vi "Format Module Name.vi"(11 "Module Path":string) -> (3 "Formatted Module Path":string)   [LabVIEW 2017, in "Routing and Faulting System Explorer.lvlib"]
uses:
  Routing and Faulting System Explorer.lvlib
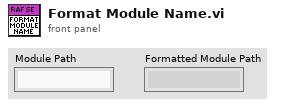
[diagram p1: front panel]
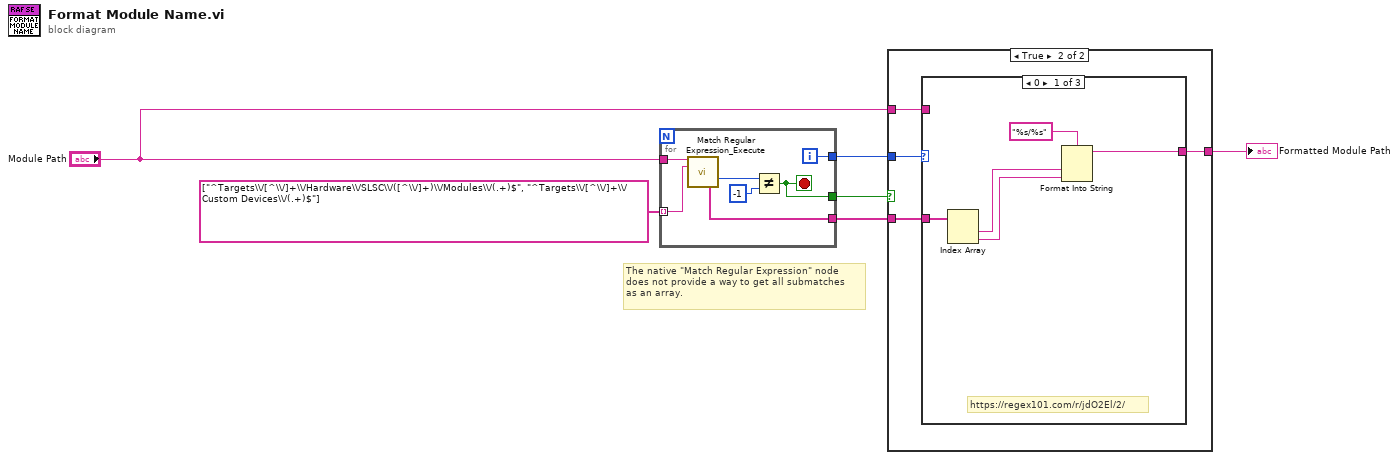
[diagram p0: block diagram]
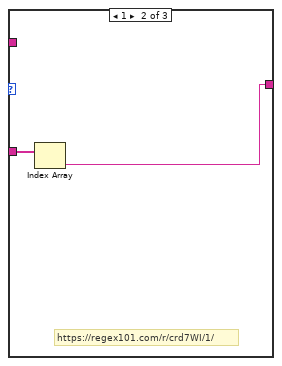
[diagram p3: hidden frame]
diagram:
  # "The native \"Match Regular Expression\" node\ndoes not provide a way to get all submatches\nas an array."
  n1 = for {
    tunnel: "Module Path" -> [w11]
    tunnel: string[] ["^Targets\\/[^\\/]+\\/Hardware\\/SLSC\\/([^\\/]+)\\/Modules\\/(.+)$", "^Targets\\/[^\\/]+\\/Custom Devices\\/(.+)$"] -> [w10] mode=indexing
    tunnel: [w12] -> w2
    tunnel: [w8] -> w4
    tunnel: [w7] -> w3
    i -> [w12]
    stop <- w7 stop-if-true
    n2 = call <vilib>:"Match Regular Expression_Execute.vi"("input string"=w11, "regular expression"=w10) -> ("whole match offset"=w9:i32, "matched substrings"=w8:string[])  [unwired: 8 in, 4 out]
    n3 = Not Equal?(x=w9, y=-1) -> (x != y?=w7:bool)
  }
  n4 = case shown="True" w3 {
    tunnel: w2 -> [_ w18]
    tunnel: w4 -> [_ w17]
    tunnel: "Module Path" -> [w14 w16]
    tunnel: [w14 w15] -> w5
    frame False {
    }
    frame True {
      n5 = case shown="0" w18 {
        tunnel: w17 -> [w23 w25 _]
        tunnel: w16 -> [_ _ w26]
        tunnel: [w19 w24 w26] -> w15
        frame 0 {
          # "https://regex101.com/r/jdO2El/2/"
          n6 = Index Array(array=w23) -> (element #1=w21:string, element #2=w20:string)  [unwired: 2 in]
          n7 = Format Into String(format string="%s/%s", w21, w20) -> (resulting string=w19:string)  [unwired: 2 in, 1 out]
        }
        frame 1 {
          # "https://regex101.com/r/crd7WI/1/"
          n8 = Index Array(array=w25) -> (element=w24:string)  [unwired: 1 in]
        }
        frame Default {
        }
      }
    }
  }
  "Formatted Module Path" <- w5
